vi "PCO_GetSizes.vi"(8 "error in (no error)":errorcluster, 11 "Handle":u64) -> (0 "error out":errorcluster, 1 "MaxRes":cluster{"wXResMax":u16, "wYResMax":u16}, 2 "ActRes":cluster{"wXResAct":u16, "wYResAct":u16}, 3 "Handle Out":u64, 5 "return type":u32 format="%x")   [LabVIEW 2011]
uses:
  SC2_Cam64.dll
panel:
  # "A00A3002 invalid Handle"
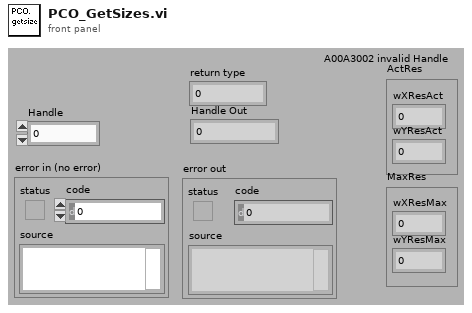
[diagram p1: front panel]
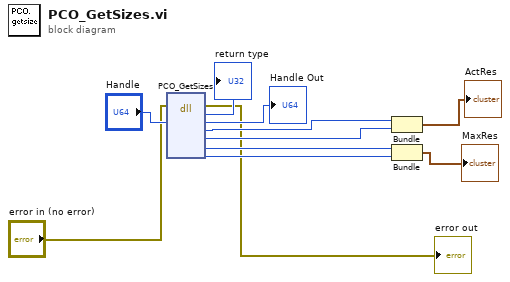
[diagram p0: block diagram]
diagram:
  n1 = dll-call lib="SC2_Cam*.*" fn="PCO_GetSizes"(error in="error in (no error)", "Handle"="Handle") -> (error out=→"error out":errorcluster, "return type"=→"return type":u32, "Handle"=→"Handle Out":u64, "wXResAct"=w8:u16, "wYResAct"=w7:u16, "wXResMax"=w5:u16, "wYResMax"=w4:u16)  [unwired: 2 in, 5 out]
  n2 = Bundle("wXResAct"=w8, "wYResAct"=w7) -> (→"ActRes":cluster{"wXResAct":u16, "wYResAct":u16})  [unwired: 1 out]
  n3 = Bundle("wXResMax"=w5, "wYResMax"=w4) -> (→"MaxRes":cluster{"wXResMax":u16, "wYResMax":u16})  [unwired: 1 out]
